vi "Local Network Timeout--Const.vi"() -> (3 "Local Network Timeout (ms)":i32)   [LabVIEW 2017, in "DTacq Plot Display Library.lvlib"]
uses:
  DTacq Plot Display Library.lvlib
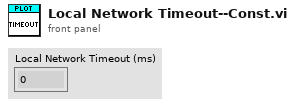
[diagram p1: front panel]
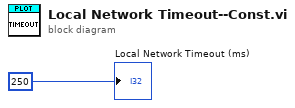
[diagram p0: block diagram]
diagram:
  "Local Network Timeout (ms)" <- 250 ("timeout ms")
